vi "Reply (varient).vi"(8 "error in (no error)":errorcluster, 9 "Varient":variant, 10 "Reply":string caption="Reply Label", 11 "Message to Reply to":refnum<class "MSG.lvclass">) -> (0 "error out":errorcluster, 3 "Message":refnum<class "MSG.lvclass">)   [LabVIEW 2011, in "Messenging.lvlib" / "MSG.lvclass"]
uses:
  MSG.lvclass
  Write VarMessage.vi
  VarMessage/VarMessage.lvclass
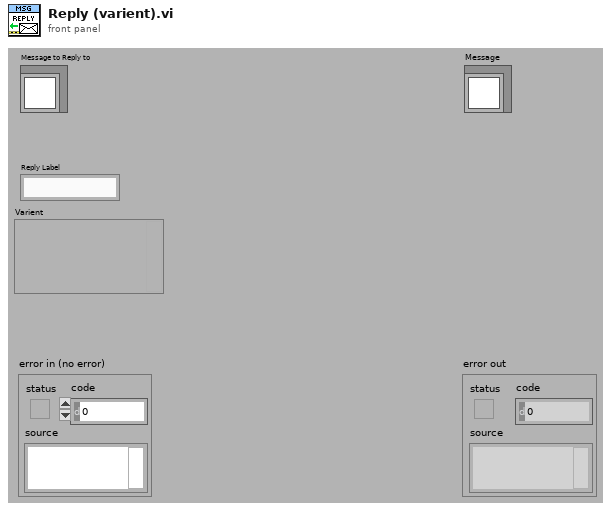
[diagram p1: front panel]
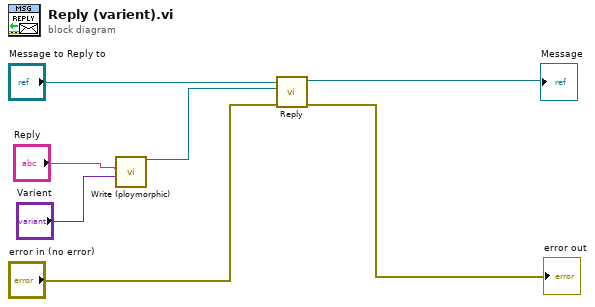
[diagram p0: block diagram]
diagram:
  n1 = call-poly "Write (ploymorphic).vi"("Varient"="Varient", "Label"="Reply") -> ("Message"=w3:refnum<class "VarMessage.lvclass">)  [unwired: 1 in, 8 out]
  n2 = call-dynamic "Reply.vi"("error in (no error)"="error in (no error)", "Reply"=w3, "Message to Reply to"="Message to Reply to") -> ("error out"=→"error out":errorcluster, "Message"=→"Message":refnum<class "MSG.lvclass">)  [unwired: 7 out]
